vi "SetText.vi"(8 "error in (no error)":errorcluster, 10 "Text":string, 11 "reference in":refnum<class "Text.lvclass">) -> (0 "error out":errorcluster, 3 "reference out":refnum<class "Text.lvclass">)   [LabVIEW 2010, in "Labricks.lvlib" / "Text.lvclass"]
uses:
  Text.lvclass
  RenderBase/SceneObject_class/SceneObject.lvclass
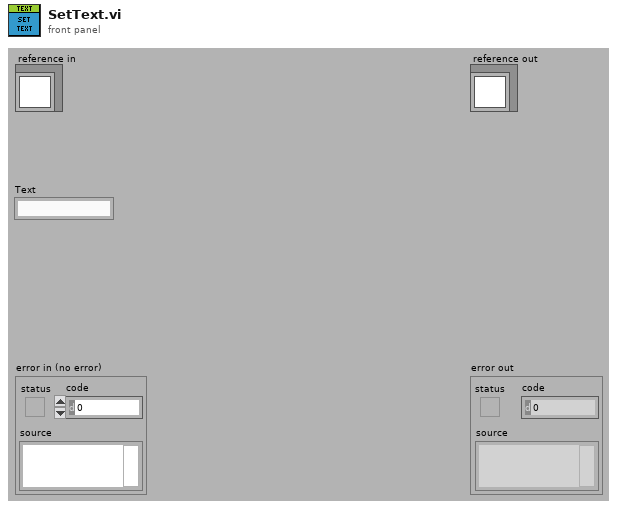
[diagram p1: front panel]
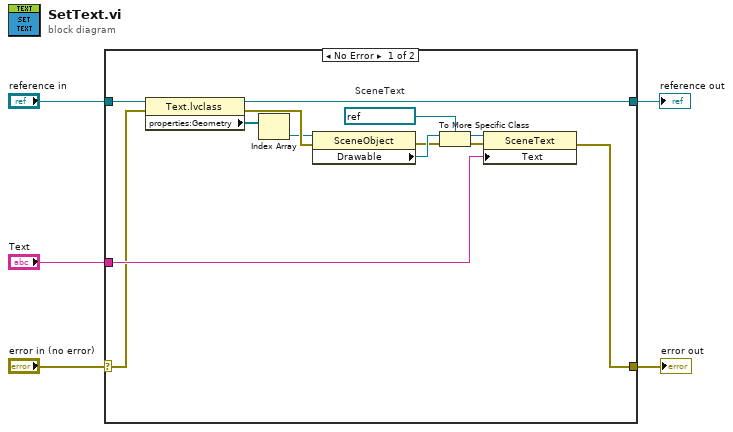
[diagram p0: block diagram]
diagram:
  n1 = case shown="No Error" "error in (no error)" {
    selector: "error in (no error)" -> [w7 w20]
    tunnel: [w9 w20] -> w4
    tunnel: [w10 w19] -> w2
    tunnel: "reference in" -> [w6 w19]
    tunnel: "Text" -> [w8 _]
    frame No Error {
      w13 = refnum<vi> refnum  # SceneText
      n2 = property class="Text.lvclass"(reference=w6, error in=w7) -> (reference out=w10:refnum<class "Text.lvclass">, error out=w16:errorcluster, "properties:Geometry"=w11:refnum<vi>[])
      n3 = Index Array(array=w11) -> (element=w12:refnum<vi>)  [unwired: 1 in]
      n4 = property class="SceneObject"(reference=w12, error in=w16) -> (error out=w17:errorcluster, "Drawable"=w18:refnum<vi>)  [unwired: 1 out]
      n5 = To More Specific Class(target class=w13, reference=w18, error in=w17) -> (specific class reference=w14:refnum<vi>, error out=w15:errorcluster)
      n6 = property class="SceneText"(reference=w14, error in=w15, "Text"=w8) -> (error out=w9:errorcluster)  [unwired: 1 out]
    }
    frame Error {
    }
  }
  "error out" <- w4
  "reference out" <- w2
